vi "XCP connect.vi"(6 "error in":errorcluster, 8 "MaxRead":i32, 9 "Channel in":u16) -> (0 "error out":errorcluster, 1 "Messages":T1(array[cluster]), 2 "Pass":bool, 3 "Channel out":u16)   [LabVIEW 2023]
uses:
  c60d9e91-3b79-4ba4-9146-ee67ae1b5e7d.vi
  Communication/PCAN2023/PCAN API.lvlib
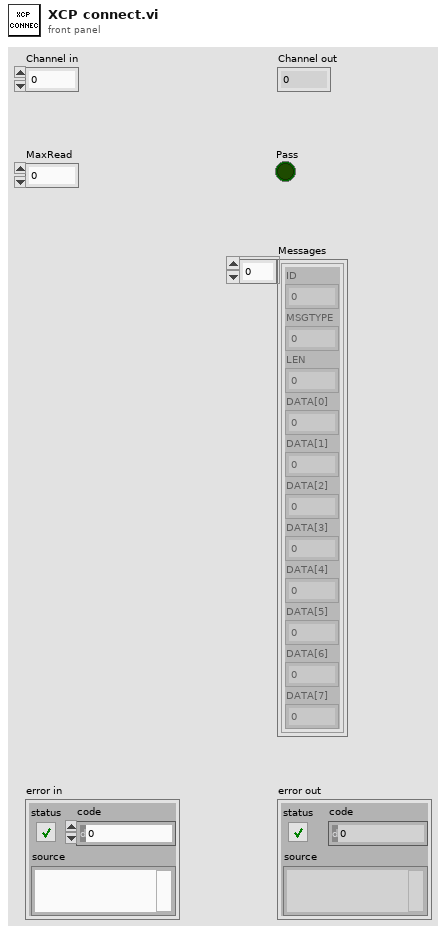
[diagram p1: front panel]
types:
  T1 = cluster{"ID":u32, "MSGTYPE":u8, "LEN":u8, "DATA[0]":u8, "DATA[1]":u8, "DATA[2]":u8, "DATA[3]":u8, "DATA[4]":u8, "DATA[5]":u8, "DATA[6]":u8, "DATA[7]":u8}[]
  T2 = cluster{"ID":u32, "MSGTYPE":u8, "LEN":u8, "DATA[0]":u8, "DATA[1]":u8, "DATA[2]":u8, "DATA[3]":u8, "DATA[4]":u8, "DATA[5]":u8, "DATA[6]":u8, "DATA[7]":u8}
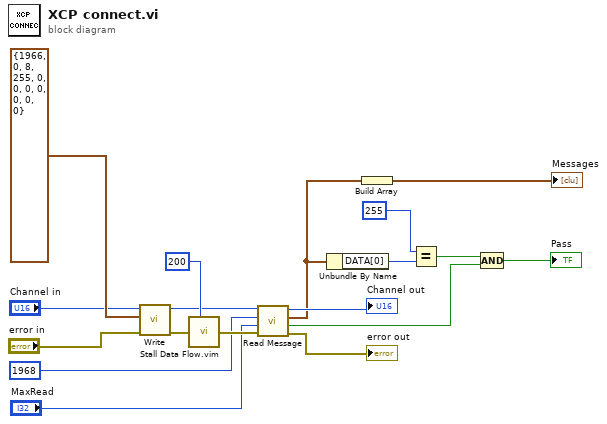
[diagram p0: block diagram]
diagram:
  n1 = call "Write.vi"("error in"="error in", "MessageBuffer"=T2 {"ID"=1966, "MSGTYPE"=0, "LEN"=8, "DATA[0]"=255, "DATA[1]"=0, "DATA[2]"=0, "DATA[3]"=0, "DATA[4]"=0, "DATA[5]"=0, "DATA[6]"=0, "DATA[7]"=0}, "Channel"="Channel in") -> ("error out"=w17:errorcluster, "Channel out"=w8:u16)  [unwired: 5 in, 2 out]
  n2 = call "Stall Data Flow.vim"("value in"=w17, "milliseconds to wait"=u32 200) -> ("value out"=w6:errorcluster)  [unwired: 1 out]
  n3 = call "Read Message.vi"("error in"=w6, "MaxRead"="MaxRead", "ID"=u32 1968, "Channel in"=w8) -> ("error out"=→"error out":errorcluster, "Passed"=w3:bool, "Last Message"=w4:T2, "Channel out"=→"Channel out":u16)  [unwired: 3 in, 1 out]
  n4 = Unbundle By Name(w4) -> ("DATA[0]"=w14:u8)
  n5 = Build Array(w4) -> (→"Messages":T1)
  n6 = Equal?(x=u8 255, y=w14) -> (x = y?=w12:bool)
  n7 = Compound Arithmetic op=AND(w12, w3) -> (→"Pass":bool)
